vi "read_log.vi"() -> ()   [LabVIEW 2013]
uses:
  cRIO_Code/Logic/Classes/Waypoint/Waypoint.lvclass
  cRIO_Code/Data/TypeDefs/Rudder Set Suggestions.ctl
  cRIO_Code/Data/TypeDefs/Sail Set Suggestions.ctl
  cRIO_Code/Data/TypeDefs/RC Input Values.ctl
  cRIO_Code/Data/TypeDefs/DynamixelCycleTracker.ctl
  cRIO_Code/Data/TypeDefs/HardwareOnline.ctl
  cRIO_Code/Data/TypeDefs/AirmarStatus.ctl
  cRIO_Code/Data/TypeDefs/DynamixelSetupInfo.ctl
  cRIO_Code/Data/TypeDefs/MotorSetup.ctl
  cRIO_Code/Data/TypeDefs/OverrideMode.ctl
  cRIO_Code/Data/TypeDefs/OverrideInformation.ctl
  cRIO_Code/Data/TypeDefs/UTM Location.ctl
  cRIO_Code/Data/TypeDefs/Notifiers.ctl
panel:
  out "latest notification":dbl
  out "value":T1
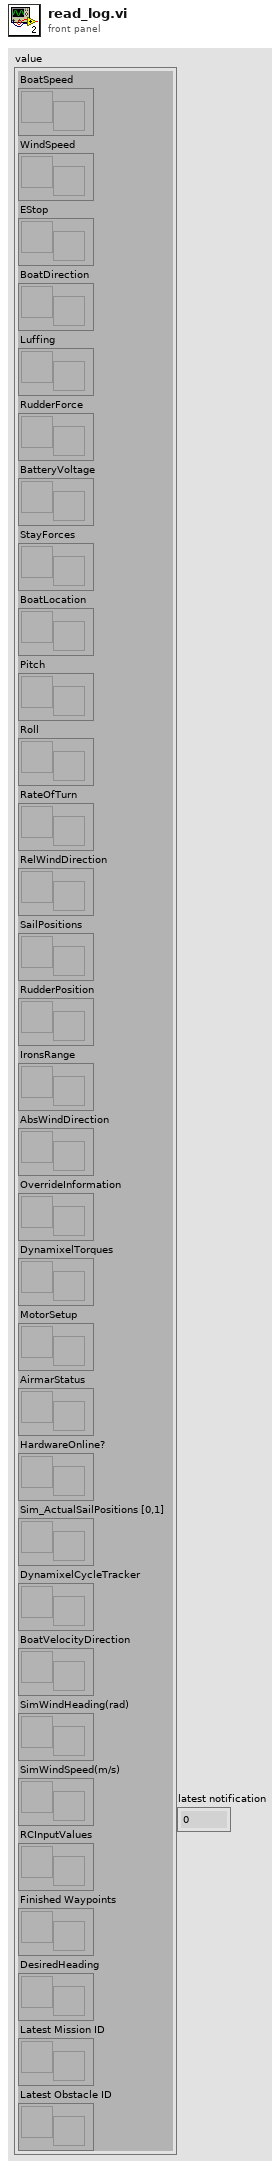
[diagram p1: front panel]
types:
  T1 = typedef "Notifiers.ctl" = cluster{"BoatSpeed":refnum<notifier>, "WindSpeed":refnum<notifier>, "EStop":refnum<notifier>, "BoatDirection":refnum<notifier>, "Luffing":refnum<notifier>, "RudderForce":refnum<notifier>, "BatteryVoltage":refnum<notifier>, "StayForces":refnum<notifier>, "BoatLocation":refnum<notifier>, "Pitch":refnum<notifier>, "Roll":refnum<notifier>, "RateOfTurn":refnum<notifier>, "RelWindDirection":refnum<notifier>, "SailPositions":refnum<notifier>, "RudderPosition":refnum<notifier>, "IronsRange":refnum<notifier>, "AbsWindDirection":refnum<notifier>, "OverrideInformation":refnum<notifier>, "DynamixelTorques":refnum<notifier>, "MotorSetup":refnum<notifier>, "AirmarStatus":refnum<notifier>, "HardwareOnline?":refnum<notifier>, "Sim_ActualSailPositions [0,1]":refnum<notifier>, "DynamixelCycleTracker":refnum<notifier>, "BoatVelocityDirection":refnum<notifier>, "SimWindHeading(rad)":refnum<notifier>, "SimWindSpeed(m/s)":refnum<notifier>, "RCInputValues":refnum<notifier>, "Finished Waypoints":refnum<notifier>, "DesiredHeading":refnum<notifier>, "Latest Mission ID":refnum<notifier>, "Latest Obstacle ID":refnum<notifier>}
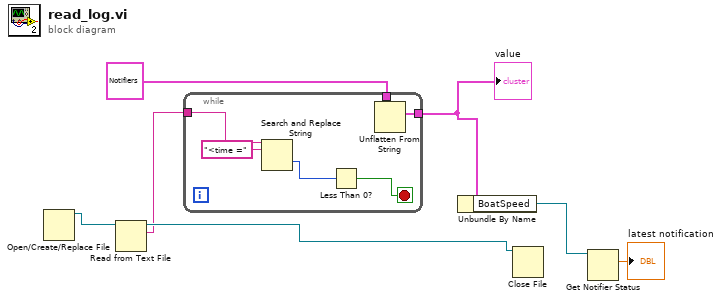
[diagram p0: block diagram]
diagram:
  n1 = Open/Create/Replace File() -> (refnum out=w7:refnum<file>)  [unwired: 6 in, 2 out]
  n2 = Read from Text File(file (use dialog)=w7) -> (refnum out=w4:refnum<file>, text=w1:string)  [unwired: 3 in, 2 out]
  n3 = while {
    tunnel: T1 {"BoatSpeed"=refnum, "WindSpeed"=refnum, "EStop"=refnum, "BoatDirection"=refnum, "Luffing"=refnum, "RudderForce"=refnum, "BatteryVoltage"=refnum, "StayForces"=refnum, "BoatLocation"=refnum, "Pitch"=refnum, "Roll"=refnum, "RateOfTurn"=refnum, "RelWindDirection"=refnum, "SailPositions"=refnum, "RudderPosition"=refnum, "IronsRange"=refnum, "AbsWindDirection"=refnum, "OverrideInformation"=refnum, "DynamixelTorques"=refnum, "MotorSetup"=refnum, "AirmarStatus"=refnum, "HardwareOnline?"=refnum, "Sim_ActualSailPositions [0,1]"=refnum, "DynamixelCycleTracker"=refnum, "BoatVelocityDirection"=refnum, "SimWindHeading(rad)"=refnum, "SimWindSpeed(m/s)"=refnum, "RCInputValues"=refnum, "Finished Waypoints"=refnum, "DesiredHeading"=refnum, "Latest Mission ID"=refnum, "Latest Obstacle ID"=refnum} ("NotifierReferences") -> [w13]
    tunnel: [w12] -> w5
    tunnel: w1 -> [w11]
    stop <- w8 stop-if-true
    n4 = Search and Replace String(input string=w11, search string="<time =") -> (offset past replacement=w9:i32)  [unwired: 6 in, 3 out]
    n5 = Less Than 0?(x=w9) -> (x < 0?=w8:bool)
    n6 = Unflatten From String(type=w13) -> (value=w12:T1)  [unwired: 4 in, 2 out]
  }
  "value" <- w5
  n7 = Unbundle By Name(w5) -> ("BoatSpeed"=w3:refnum<notifier>)
  n8 = Close File(refnum=w4) -> ()  [unwired: 1 in, 2 out]
  n9 = Get Notifier Status(notifier=w3) -> (current notification=→"latest notification":dbl)  [unwired: 1 in, 4 out]
